vi "Set_PreviewCache.vi"(8 "error in (no error)":errorcluster, 10 "data":T1, 11 "PreviewCache in":refnum<class "PreviewCache.lvclass">) -> (0 "error out":errorcluster, 3 "PreviewCache out":refnum<class "PreviewCache.lvclass">)   [LabVIEW 2020, in "PreviewCache.lvclass"]
uses:
  <vilib>/AppBuilder/AB_Classes/PreviewCache/PreviewCache.lvclass
  <vilib>/AppBuilder/AB_Classes/PreviewCache/PreviewCache.ctl
  <vilib>/AppBuilder/AB_Classes/PreviewCache/build preview data.ctl
  <vilib>/AppBuilder/AB_Classes/PreviewCache/PreviewCache.lvclass/PreviewCache.ctl
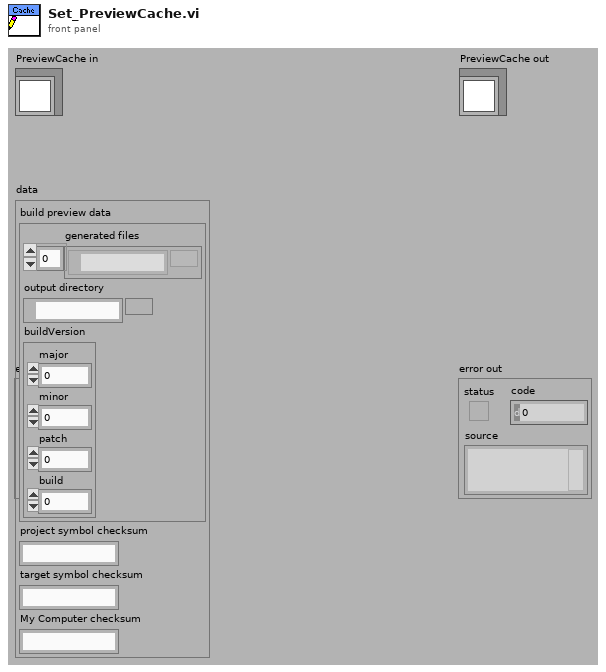
[diagram p1: front panel]
types:
  T1 = typedef "PreviewCache.ctl" = cluster{"build preview data":T2, "project symbol checksum":string, "target symbol checksum":string, "My Computer checksum":string}
  T2 = typedef "build preview data.ctl" = cluster{"generated files":path[], "output directory":path, "buildVersion":cluster{"major":u16, "minor":u16, "patch":u16, "build":u16}}
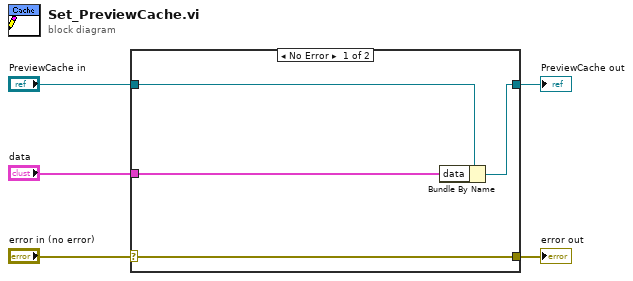
[diagram p0: block diagram]
diagram:
  n1 = case shown="No Error" "error in (no error)" {
    selector: "error in (no error)" -> [w9 w10]
    tunnel: [w9 w10] -> w4
    tunnel: [w7 w11] -> w2
    tunnel: "PreviewCache in" -> [w8 w11]
    tunnel: "data" -> [w6 _]
    frame No Error {
      n2 = Bundle By Name(cluster=w8, "data"=w6) -> (w7:refnum<class "PreviewCache.lvclass">)
    }
    frame Error {
    }
  }
  "error out" <- w4
  "PreviewCache out" <- w2
